vi "Modulus2D.vi"(8 "error in (no error)":errorcluster, 10 "2D vector":dbl[](array[numeric]), 11 "Utilities in":refnum<class "Utilities.lvclass">) -> (0 "error out":errorcluster, 2 "Modulus":dbl, 3 "Utilities out":refnum<class "Utilities.lvclass">)   [LabVIEW 2018, in "Utilities.lvclass"]
uses:
  Utilities.lvclass
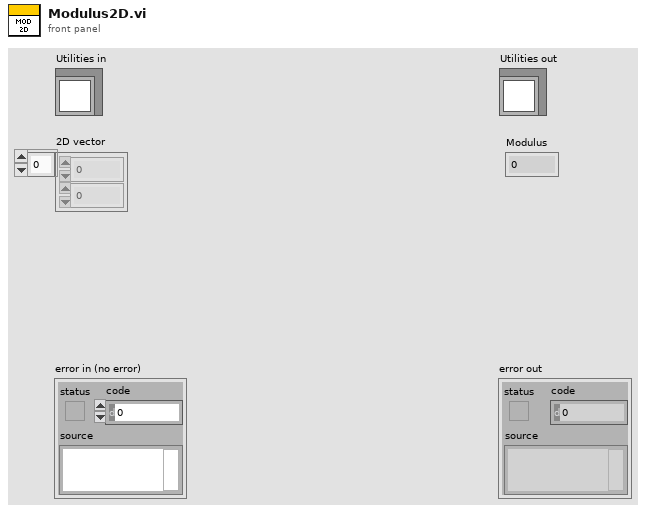
[diagram p1: front panel]
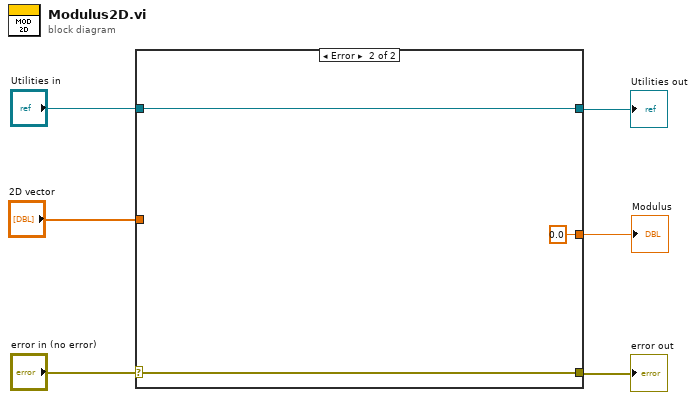
[diagram p0: block diagram]
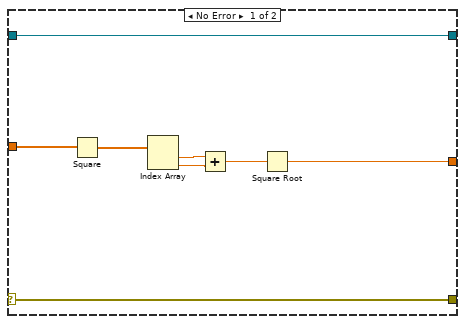
[diagram p2: hidden frame]
diagram:
  n1 = case shown="Error" "error in (no error)" {
    selector: "error in (no error)" -> [w13 w17]
    tunnel: [w13 w17] -> w5
    tunnel: [w14 w16] -> w3
    tunnel: "Utilities in" -> [w14 w16]
    tunnel: "2D vector" -> [w8 _]
    tunnel: [w7 0.0] -> w1
    frame No Error {
      n2 = Square(x=w8) -> (x^2=w9:dbl[])
      n3 = Index Array(array=w9) -> (element #1=w10:dbl, element #2=w11:dbl)  [unwired: 2 in]
      n4 = Add(x=w10, y=w11) -> (x+y=w12:dbl)
      n5 = Square Root(x=w12) -> (sqrt(x)=w7:dbl)
    }
    frame Error {
    }
  }
  "error out" <- w5
  "Utilities out" <- w3
  "Modulus" <- w1
